vi "3.11-Pick Most Important Point.vi"(1 "Old Point":T1, 2 "New Point":T1, 3 "Side":enum16{"Left", "Right"}(ring)) -> (0 "Most Limiting Point":T1)   [LabVIEW 2011]
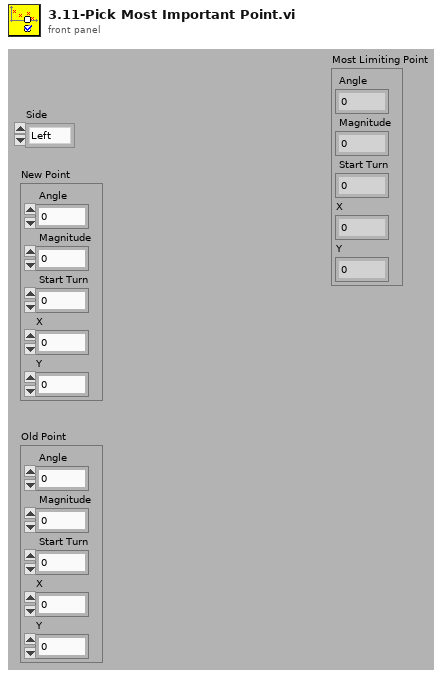
[diagram p1: front panel]
types:
  T1 = cluster{" Angle":dbl, " Magnitude":dbl, " Start Turn":dbl, "X":dbl, "Y":dbl}
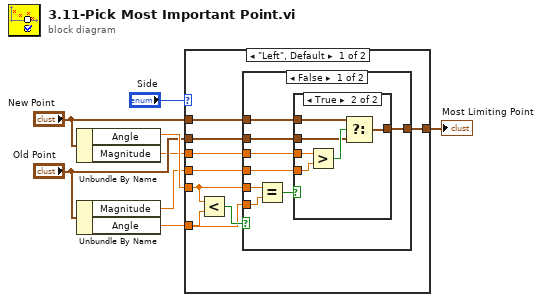
[diagram p0: block diagram]
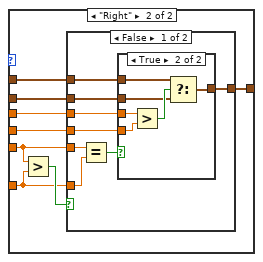
[diagram p4: hidden frame]
diagram:
  n1 = Unbundle By Name("New Point") -> ("Angle"=w7:dbl, "Magnitude"=w2:dbl)
  n2 = Unbundle By Name("Old Point") -> ("Magnitude"=w1:dbl, "Angle"=w6:dbl)
  n3 = case shown="\"Left\", Default" "Side" {
    tunnel: w7 -> [w9 w37]
    tunnel: w6 -> [w10 w36]
    tunnel: [w14 w39] -> w4
    tunnel: "New Point" -> [w16 w38]
    tunnel: "Old Point" -> [w15 w35]
    tunnel: w2 -> [w13 w34]
    tunnel: w1 -> [w12 w33]
    frame "Left", Default {
      n4 = Less?(x=w9, y=w10) -> (x < y?=w11:bool)
      n5 = case shown="False" w11 {
        tunnel: [w21 w32] -> w14
        tunnel: w16 -> [w17 w32]
        tunnel: w9 -> [w24 _]
        tunnel: w10 -> [w23 _]
        tunnel: w15 -> [w20 _]
        tunnel: w13 -> [w19 _]
        tunnel: w12 -> [w18 _]
        frame False {
          n6 = Equal?(x=w24, y=w23) -> (x = y?=w22:bool)
          n7 = case shown="True" w22 {
            tunnel: [w25 w26] -> w21
            tunnel: w20 -> [w25 w27]
            tunnel: w19 -> [_ w30]
            tunnel: w18 -> [_ w29]
            tunnel: w17 -> [_ w28]
            frame False {
            }
            frame True {
              n8 = Greater?(x=w30, y=w29) -> (0:w31:bool)
              n9 = Select(t=w28, s=w31, f=w27) -> (s? t:f=w26:T1)
            }
          }
        }
        frame True {
        }
      }
    }
    frame "Right" {
      n10 = Greater?(x=w37, y=w36) -> (0:w40:bool)
      n11 = case shown="False" w40 {
        tunnel: [w45 w56] -> w39
        tunnel: w38 -> [w41 w56]
        tunnel: w37 -> [w48 _]
        tunnel: w36 -> [w47 _]
        tunnel: w35 -> [w44 _]
        tunnel: w34 -> [w43 _]
        tunnel: w33 -> [w42 _]
        frame False {
          n12 = Equal?(x=w48, y=w47) -> (x = y?=w46:bool)
          n13 = case shown="True" w46 {
            tunnel: [w49 w50] -> w45
            tunnel: w44 -> [w49 w51]
            tunnel: w43 -> [_ w54]
            tunnel: w42 -> [_ w53]
            tunnel: w41 -> [_ w52]
            frame False {
            }
            frame True {
              n14 = Greater?(x=w54, y=w53) -> (0:w55:bool)
              n15 = Select(t=w52, s=w55, f=w51) -> (s? t:f=w50:T1)
            }
          }
        }
        frame True {
        }
      }
    }
  }
  "Most Limiting Point" <- w4
